vi "ang.vi"(8 "에러 입력":errorcluster, 9 "spring pull":dbl, 10 "wanted angle":dbl, 11 "FPGA VI 참조 입력":refnum<k20>) -> (0 "에러 출력":errorcluster, 2 "대포를 다 쏨????":bool, 3 "FPGA VI 참조 출력":refnum<k20>)   [LabVIEW 2019]
uses:
  <vilib>/Platform/TimedLoop/XDataNode/timing_clust.ctl
  <vilib>/Platform/TimedLoop/XDataNode/nitl_modes.ctl
  <vilib>/Platform/TimedLoop/XDataNode/wakeup.ctl
  <vilib>/Utility/error.llb/Error Cluster From Error Code.vi
  <vilib>/rvi/errors/niLvFpgaAdjustHostInterfaceError.vi
  <vilib>/rvi/interface/nirviReadWriteControl/nirviReadWriteControl.xnode
  <vilib>/Platform/TimedLoop/XDataNode/XDataNode.xnode
  <vilib>/Platform/TimedLoop/XDataNode/XDNodeRunTimeDep.lvlib
  <vilib>/rvi/interface/Simulation/niFpgaSimulationCallBeginRW.vi
  NiFpgaLv.dll
panel:
  out "숫자형":i32
  in  "정지":bool
  out "reference":cluster{"wanted angle":dbl, dbl}(graph)={"wanted angle"=-36.7, 0.0}
  in  "Ki":dbl=50.0
  in  "Kd":dbl=0.01
  out "방향":bool
  out "u(k) = pwm":dbl
  in  "Kp":dbl=500.0
  out "now angle":dbl
  out "Now mot rev":dbl
  out "Timeout":i32
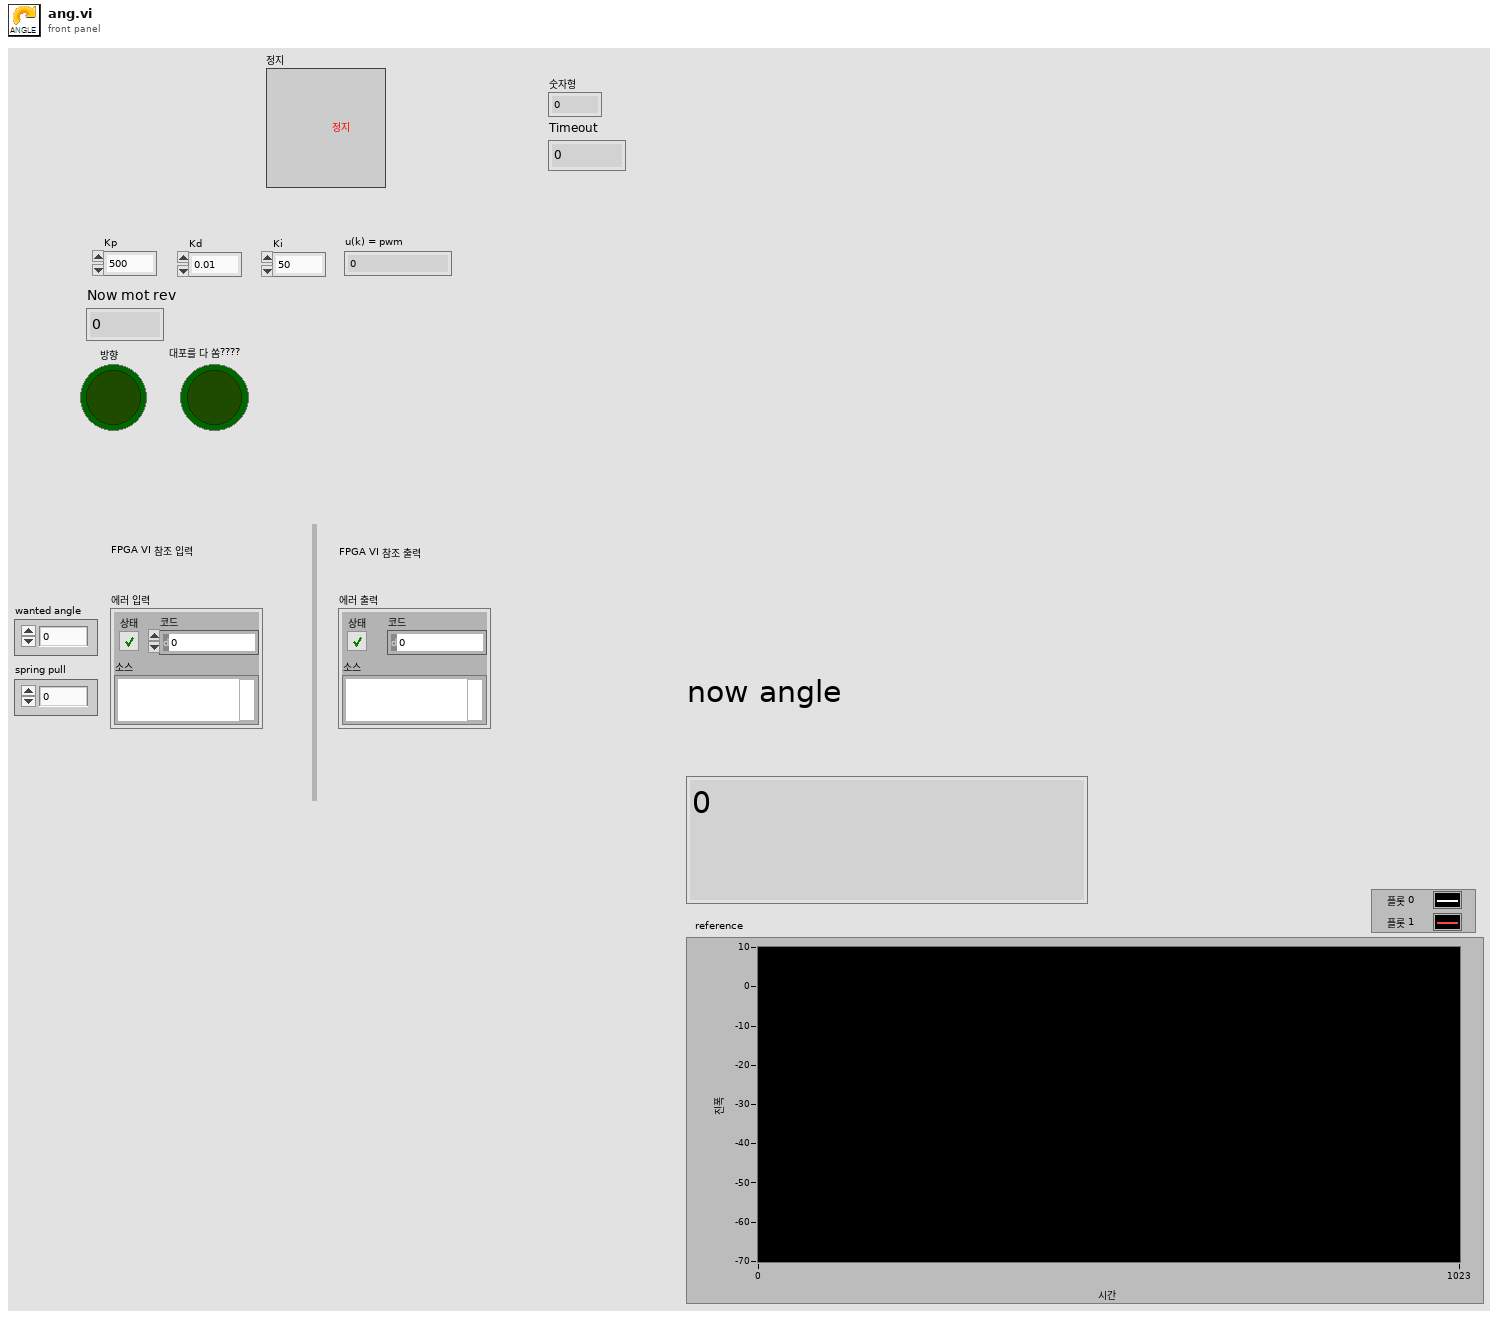
[diagram p1: front panel]
types:
  T1 = typedef "XDNodeRunTimeDep.lvlib/timing_clust.ctl" = cluster{"Expected End [f-1]":u64, "Actual End [f-1]":u64, "Finished Late? [f-1]":bool, "Expected End [i-1]":u64, "Actual End [i-1]":u64, "Finished Late? [i-1]":bool, "Expected Start [i]":u64, "Actual Start [i]":u64, "Expected Start [f]":u64, "Actual Start [f]":u64, "Source Name":string, "Structure Name":string, "Period":i64, "Deadline":i64, "Offset":i64, "Start":i64, "Priority":i32, "Timeout":i32, "Mode":T2, "Wakeup Reason":T3, "Error":errorcluster, "Source Type":string, "Secondary Source Type":string, "Global End Time":u64, "Global Start Time":u64, "Frame Duration":u64, "Iteration Duration":u64, "Assigned CPU":i32, "I/O Scan Engine Mode":u32}
  T2 = typedef "XDNodeRunTimeDep.lvlib/nitl_modes.ctl" = enum32{"No Change", "Process missed periods, maintain original phase", "Discard missed periods, maintain original phase", "Process missed periods, ignore original phase", "Discard missed periods, ignore original phase"}
  T3 = typedef "XDNodeRunTimeDep.lvlib/wakeup.ctl" = enum32{"Normal", "Aborted", "Asynchronous wakeup", "Timing source error", "Timed loop error", "Timeout"}
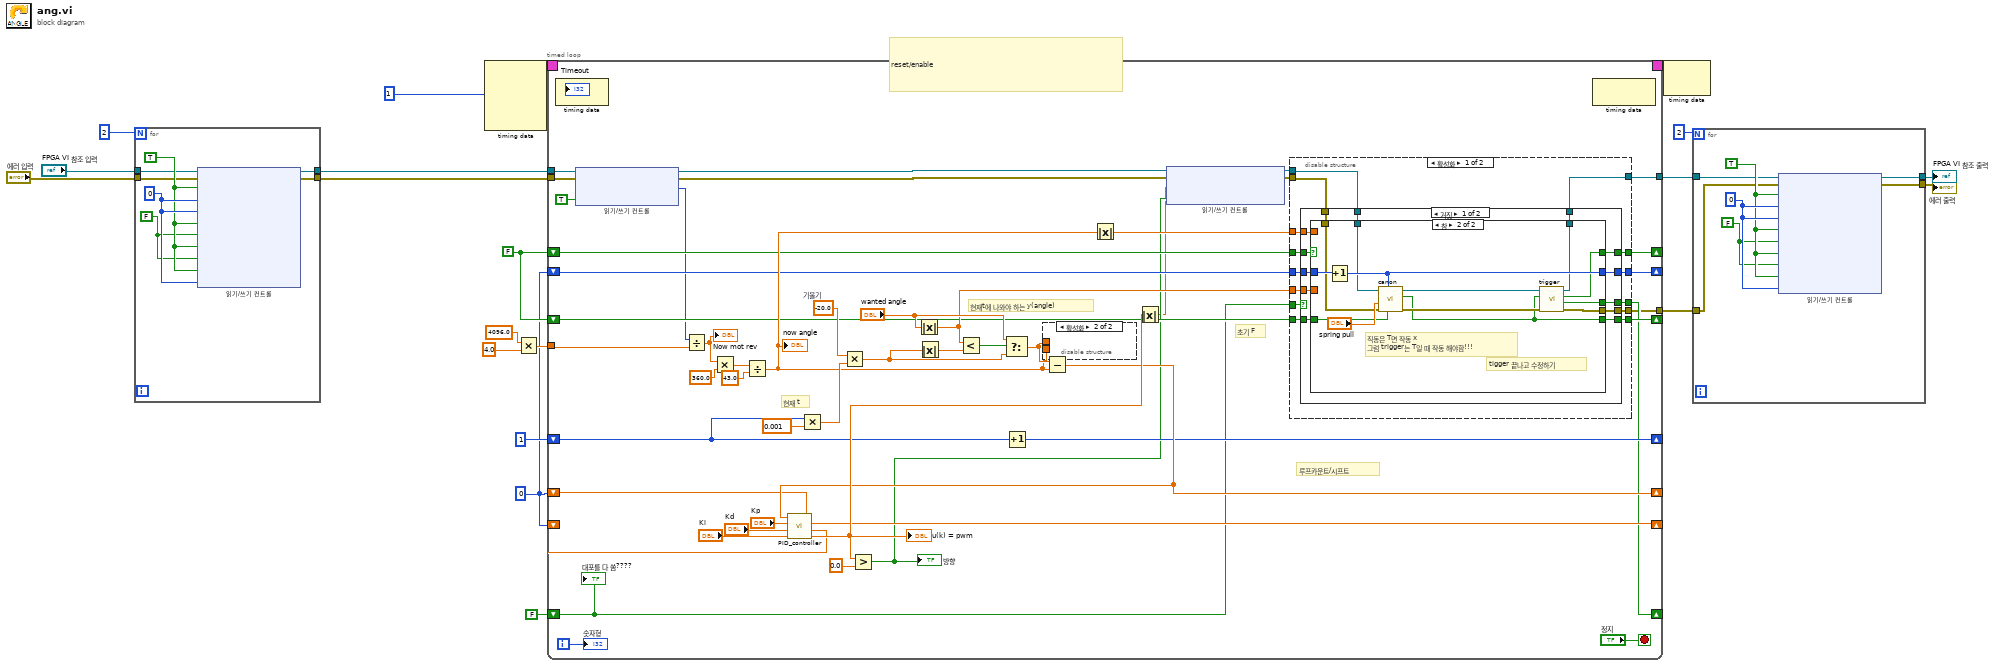
[diagram p0: block diagram]
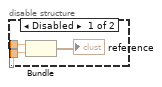
[diagram p2: hidden frame]
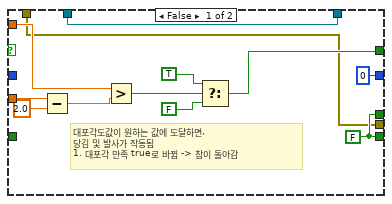
[diagram p3: hidden frame]
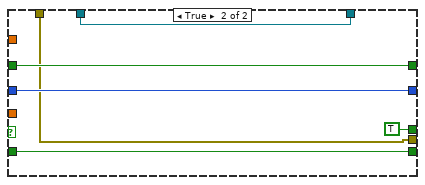
[diagram p4: hidden frame]
diagram:
  w12 = FALSE ("encoder reset")
  w11 = 0
  # "reset/enable"
  n1 = for {
    N: 2 -> [_]
    tunnel: [w24] -> w9
    tunnel: [w23] -> w8
    tunnel: "FPGA VI 참조 입력" -> [w22]
    tunnel: "에러 입력" -> [w21]
    w26 = TRUE ("encoder reset")
    w25 = FALSE ("encoder reset")
    w27 = 0 ("Encoder  (4x)")
    n2 = xnode "읽기/쓰기 컨트롤"("FPGA VI 참조 입력"=w22, "에러 입력"=w21, "encoder reset"=w26, "pwm input"=w27, "직동_pwm input"=w27, "angle_encoder reset"=w26, "angle_Enable (escon)"=w25, "tir_encoder reset"=w26, "tir_Enable (escon)"=w25, "R_encoder reset"=w26, "R_pwm input"=w27) -> ("FPGA VI 참조 출력"=w24:refnum<k20>, "에러 출력"=w23:errorcluster)
  }
  n3 = node-c288(i64 1 ("주기")) -> (w20:T1)  [unwired: 3 in]
  n4 = Multiply(x=4096.0, y=4.0) -> (x*y=w15:dbl)
  n5 = timed-loop {
    timing: w20 -> [_]
    timing-out: [_] -> w19
    tunnel: w15 -> [w54]
    shift-right: [w59] -> _
    shift-left: 1 -> [w57]
    shift-right: [w60] -> _
    shift-left: w11 -> [w56]
    shift-right: [w58] -> _
    shift-left: w11 -> [w55]
    shift-right: [w50] -> _
    shift-left: w12 -> [w49]
    shift-right: [w46] -> _
    shift-left: w12 -> [w45]
    shift-right: [w43] -> _
    shift-left: w11 -> [w44]
    shift-right: [w41] -> _
    shift-left: FALSE ("대포를 다 쏘았나용????") -> [w42]
    tunnel: w9 -> [w39]
    tunnel: w8 -> [w38]
    tunnel: [w29] -> w7
    tunnel: [w28] -> w6
    i -> [w40]
    stop <- "정지" stop-if-true
    w71 = -20.0  # 기울기
    # "초기 F"
    # "루프카운트/시프트"
    # "현재t에 나와야 하는 y(angle)"
    # "현재 t"
    n6 = node-c288() -> (→"Timeout":i32)  [unwired: 1 in]
    n7 = xnode "읽기/쓰기 컨트롤"("FPGA VI 참조 입력"=w39, "에러 입력"=w38, "angle_Enable (escon)"=TRUE ("encoder reset")) -> ("FPGA VI 참조 출력"=w35:refnum<k20>, "에러 출력"=w34:errorcluster, "angle_Encoder  (4x)"=w36:i32)
    n8 = Divide(x=w36, y=w54) -> (x/y=w74:dbl)
    "Now mot rev" <- w74
    n9 = Multiply(x=w74, y=360.0) -> (x*y=w62:dbl)
    n10 = Divide(x=w62, y=43.0) -> (x/y=w51:dbl)
    "now angle" <- w51
    n11 = Multiply(x=w57, y=0.001) -> (x*y=w69:dbl)
    n12 = Multiply(x=w71, y=w69) -> (x*y=w64:dbl)
    n13 = Absolute Value(x="wanted angle") -> (abs(x)=w47:dbl)
    n14 = Absolute Value(x=w64) -> (abs(x)=w63:dbl)
    n15 = Less?(x=w47, y=w63) -> (x < y?=w68:bool)
    n16 = Select(t="wanted angle", s=w68, f=w64) -> (s? t:f=w61:dbl)
    n17 = Increment(x=w57) -> (x+1=w59:i32)
    n18 = disable-structure shown="활성화" {
      disable-tunnel: w61 -> [w80 _]
      disable-tunnel: w51 -> [w78 _]
      frame Disabled {
        n19 = Bundle("wanted angle"=w80, w78) -> (→"reference":cluster{"wanted angle":dbl, dbl})  [unwired: 1 in]
      }
      frame Enabled {
      }
    }
    n20 = Subtract(x=w61, y=w51) -> (x-y=w60:dbl)
    n21 = call "PID_controller.vi"("Error_Sum(k-1)"=w55, "Error(k-1)"=w56, "Ki"="Ki", "Kd"="Kd", "Kp"="Kp", "Error(k)"=w60) -> ("u(k)"=w67:dbl, "Error_Sum(k)"=w58:dbl)
    "u(k) = pwm" <- w67
    n22 = Greater?(x=w67, y=0.0) -> (0:w33:bool)
    "방향" <- w33
    n23 = Absolute Value(x=w51) -> (abs(x)=w48:dbl)
    n24 = Absolute Value(x=w67) -> (abs(x)=w32:dbl)
    n25 = xnode "읽기/쓰기 컨트롤"("FPGA VI 참조 입력"=w35, "에러 입력"=w34, "angle_pwm input(escon)"=w32, "angle_DIR"=w33) -> ("FPGA VI 참조 출력"=w31:refnum<k20>, "에러 출력"=w30:errorcluster)
    n26 = disable-structure shown="활성화" {
      disable-tunnel: [w94 w142] -> w50
      disable-tunnel: w49 -> [w93 w142]
      disable-tunnel: w48 -> [w92 _]
      disable-tunnel: w47 -> [w91 _]
      disable-tunnel: w31 -> [w84 w144]
      disable-tunnel: w30 -> [w83 w143]
      disable-tunnel: [w90 w140] -> w46
      disable-tunnel: w45 -> [w89 w140]
      disable-tunnel: w44 -> [w88 w139]
      disable-tunnel: [w87 w139] -> w43
      disable-tunnel: w42 -> [w86 w141]
      disable-tunnel: [w85 w141] -> w41
      disable-tunnel: [w82 _] -> w29
      disable-tunnel: [w81 _] -> w28
      frame Enabled {
        n27 = case shown="거짓" w86 {
          tunnel: [w107 w137] -> w94
          tunnel: w93 -> [w106 w137]
          tunnel: w92 -> [w105 _]
          tunnel: w91 -> [w104 _]
          tunnel: [w103 w138] -> w90
          tunnel: w89 -> [w102 w138]
          tunnel: w88 -> [w101 w136]
          tunnel: [w100 w136] -> w87
          tunnel: [w99 TRUE ("대포를 다 쏘았나용????")] -> w85
          tunnel: w84 -> [w98 w134]
          tunnel: w83 -> [w97 w133]
          tunnel: [w96 w134] -> w82
          tunnel: [w95 w133] -> w81
          frame False {
            n28 = case shown="참" w106 {
              tunnel: [w119 w125] -> w107
              tunnel: w105 -> [w115 _]
              tunnel: w104 -> [w110 _]
              tunnel: [w113 w126] -> w103
              tunnel: w102 -> [_ w129]
              tunnel: w101 -> [_ w128]
              tunnel: [0 w127] -> w100
              tunnel: [w113 w124] -> w99
              tunnel: w98 -> [w111 w123]
              tunnel: w97 -> [w112 w122]
              tunnel: [w111 w121] -> w96
              tunnel: [w112 w120] -> w95
              frame False {
                w113 = FALSE ("encoder reset")
                # "대포각도값이 원하는 값에 도달하면,\n당김 및 발사가 작동됨\n1. 대포각 만족 true로 바뀜 -> 참이 돌아감"
                n29 = Subtract(x=w110, y=2.0) -> (x-y=w109:dbl)
                n30 = Greater?(x=w115, y=w109) -> (0:w116:bool)
                n31 = Select(t=TRUE ("encoder reset"), s=w116, f=FALSE ("encoder reset")) -> (s? t:f=w119:bool)
              }
              frame True {
                # "tigger 끝나고 수정하기"
                # "직동은 T면 작동 x\n그럼 trigger는 T일 때 작동 해야함!!!"
                n32 = Increment(x=w128) -> (x+1=w127:i32)
                n33 = call "canon.vi"("T/F"=w129, "loop count"=w127, "에러 입력"=w122, "spring pull[mm]"="spring pull", "FPGA VI 참조 입력"=w123) -> ("에러 출력"=w131:errorcluster, "직동_dir"=w126:bool, "FPGA VI 참조 출력"=w132:refnum<k20>)  [unwired: 4 in]
                n34 = call "trigger.vi"("에러 입력"=w131, "불리언"=w126, "FPGA VI 참조 입력"=w132) -> ("에러 출력"=w120:errorcluster, "대포발사 Y/N"=w124:bool, "불리언 2"=w125:bool, "FPGA VI 참조 출력"=w121:refnum<k20>)  [unwired: 5 in]
              }
            }
          }
          frame True {
          }
        }
      }
      frame Disabled {
      }
    }
    n35 = node-c288() -> ()  [unwired: 1 in, 1 out]
    "숫자형" <- w40
    "대포를 다 쏨????" <- w42
  }
  n36 = node-c288(w19) -> ()  [unwired: 1 out]
  n37 = for {
    N: 2 -> [_]
    tunnel: [w151] -> w3
    tunnel: [w150] -> w2
    tunnel: w7 -> [w149]
    tunnel: w6 -> [w148]
    w153 = TRUE ("encoder reset")
    w152 = FALSE ("encoder reset")
    w154 = 0 ("Encoder  (4x)")
    n38 = xnode "읽기/쓰기 컨트롤"("FPGA VI 참조 입력"=w149, "에러 입력"=w148, "encoder reset"=w153, "pwm input"=w154, "직동_pwm input"=w154, "angle_encoder reset"=w153, "angle_Enable (escon)"=w152, "tir_encoder reset"=w153, "tir_Enable (escon)"=w152, "R_encoder reset"=w153, "R_pwm input"=w154) -> ("FPGA VI 참조 출력"=w151:refnum<k20>, "에러 출력"=w150:errorcluster)
  }
  "FPGA VI 참조 출력" <- w3
  "에러 출력" <- w2
